vi "follow_angle.vi"() -> (3 "PID A":T2(graph)={"Setpoint"=-0.02930742489899981, "output"=0.018032836156553524, "dx/dt"=0.0})   [LabVIEW 2017]
uses:
  <vilib>/myRIO/Common/Instrument Driver Framework/myRIO v1.0/Encoder/typedefs/Encoder Signal Mode.ctl
  <vilib>/myRIO/Instrument Drivers/Onboard IO/Encoder/typedefs/Encoder Reference.ctl
  <vilib>/myRIO/Common/Instrument Driver Framework/Utilities/typedefs/myRIO Generic Hardware Reference.ctl
  <vilib>/myRIO/Common/Instrument Driver Framework/Utilities/typedefs/Hardware Version Enum.ctl
  <vilib>/myRIO/Common/Instrument Driver Framework/Utilities/typedefs/myRIO v1.0 Reference.ctl
  <vilib>/myRIO/Common/Instrument Driver Framework/Utilities/typedefs/Generic FPGA Reference.ctl
  <vilib>/myRIO/Common/Instrument Driver Framework/myRIO v1.0/Encoder/typedefs/Encoder Channels Enum.ctl
  <vilib>/myRIO/Common/Instrument Driver Framework/myRIO v1.0/Encoder/typedefs/Encoder Configuration v1.0.ctl
  <vilib>/userdefined/High Color/nirio_resource_hc.ctl
  <vilib>/myRIO/Common/Instrument Driver Framework/Utilities/vis/Is FPGA Ref Available.vi
  <vilib>/myRIO/Common/Instrument Driver Framework/myRIO v1.0/Encoder/vis/myRIO v1.1 Open Encoder.vi
  <vilib>/myRIO/Instrument Drivers/Onboard IO/Encoder/vis/Read.vi
  <vilib>/myRIO/Common/Instrument Driver Framework/Utilities/vis/Validate Channels.vi
  <vilib>/myRIO/Common/Instrument Driver Framework/myRIO v1.0/Encoder/vis/myRIO v1.0 Reserve Encoder.vi
  <vilib>/myRIO/Common/Instrument Driver Framework/myRIO v1.0/UART/vis/myRIO v1.0 Close UART.vi
  <vilib>/myRIO/Common/Instrument Driver Framework/myRIO v1.0/Encoder/vis/myRIO v1.0 Build MUX Configuration Encoder.vi
  <vilib>/myRIO/Common/Instrument Driver Framework/myRIO v1.0/Resource Manager/vis/myRIO v1.0 Reserve Channel List.vi
  <vilib>/myRIO/Common/Instrument Driver Framework/myRIO v1.0/Resource Manager/vis/myRIO v1.0 Create Configuration List.vi
  <vilib>/myRIO/Common/Instrument Driver Framework/myRIO v1.0/Resource Manager/vis/myRIO v1.0 Reserve Channel.vi
  <vilib>/myRIO/Common/Instrument Driver Framework/myRIO v1.0/Resource Manager/vis/myRIO v1.0 Unreserve Channel.vi
  <vilib>/myRIO/Common/Instrument Driver Framework/myRIO v1.0/Resource Manager/vis/myRIO v1.0 Build Mutex Name.vi
  <vilib>/Utility/VariantDataType/GetNumericInfo.vi
  <vilib>/Utility/error.llb/Error Cluster From Error Code.vi
  <vilib>/myRIO/Common/Instrument Driver Framework/myRIO v1.0/myRIO v1.1 Open.vi
  <vilib>/myRIO/Common/Instrument Driver Framework/Utilities/vis/IO Manager.vi
  <vilib>/myRIO/Common/Instrument Driver Framework/Utilities/vis/Configuration Manager.vi
  <vilib>/myRIO/Common/Instrument Driver Framework/myRIO v1.0/Resource Manager/vis/myRIO v1.0 Configure IO.vi
  <vilib>/myRIO/Common/Instrument Driver Framework/myRIO v1.0/myRIO v1.0 Close.vi
  <vilib>/myRIO/Common/Instrument Driver Framework/myRIO v1.0/Encoder/vis/myRIO v1.0 Configure Encoder.vi
  <vilib>/myRIO/Common/Instrument Driver Framework/myRIO v1.0/Encoder/vis/myRIO v1.0 Read Encoder.vi
  <vilib>/myRIO/Common/Instrument Driver Framework/Utilities/vis/FPGA Ref Manager.vi
  <vilib>/myRIO/Common/Instrument Driver Framework/myRIO v1.0/myRIO v1.0 Reset FPGA.vi
  <vilib>/myRIO/Common/Instrument Driver Framework/myRIO v1.0/IRQ/vis/myRIO v1.0 IRQ Info FGV.vi
  <vilib>/myRIO/Common/Instrument Driver Framework/myRIO v1.0/IRQ/vis/myRIO v1.0 Timer IRQ Info FGV.vi
  <vilib>/myRIO/Common/Instrument Driver Framework/myRIO v1.0/IRQ/vis/myRIO v1.0 ISR Agent.vi
  <vilib>/addons/control/pid/pid.llb/PID (DBL).vi
  <vilib>/myRIO/Express VI/Onboard IO/Encoder/Encoder Express VI.xnode
  <vilib>/myRIO/Instrument Drivers/Onboard IO/Encoder/vis/myRIO Encoder Open.xnode
  <vilib>/myRIO/Common/Instrument Driver Framework/myRIO v1.0/Encoder/typedefs/Encoder Count Direction Enum.ctl
  <vilib>/myRIO/Instrument Drivers/Utilities/Utilities.lvlib
  <vilib>/myRIO/Instrument Drivers/Onboard IO/Encoder/Encoder.lvlib
  <vilib>/addons/control/pid/NI_PID_pid.lvlib
panel:
  out "Angle":cluster{"Angle to Follow":dbl, dbl}(graph)={"Angle to Follow"=-9.27038626609442, -9.052560000004503}
  in  "Angle PIDS":T1={"proportional gain (Kc)"=0.05, "integral time (Ti, min)"=0.05, "derivative time (Td, min)"=0.0} {"derivative time (Td, min)" format="%.3f"; "integral time (Ti, min)" format="%.3f"; "proportional gain (Kc)" format="%.3f"}
  in  "Angle to Follow":dbl(slide)=-9.27038626609442 scale=-360.0..360.0
  in  "stop":bool
  in  "Speed":dbl(slide)=-0.015174506828527612 scale=-10.0..10.0
  out "OUTPUT B":dbl(slide) scale=-10.0..10.0
  out "OUTPUT A":dbl(slide) scale=-10.0..10.0
  out "PID B":T2(graph)={"Setpoint"=-0.0010415887580554149, "output"=-0.02086159598615355, "dx/dt"=0.0}
  out "Setpoint A":dbl(slide)=-0.02930742489899981 scale=-10.0..10.0
  out "Setpoint B":dbl(slide)=-0.0010415887580554149 scale=-10.0..10.0
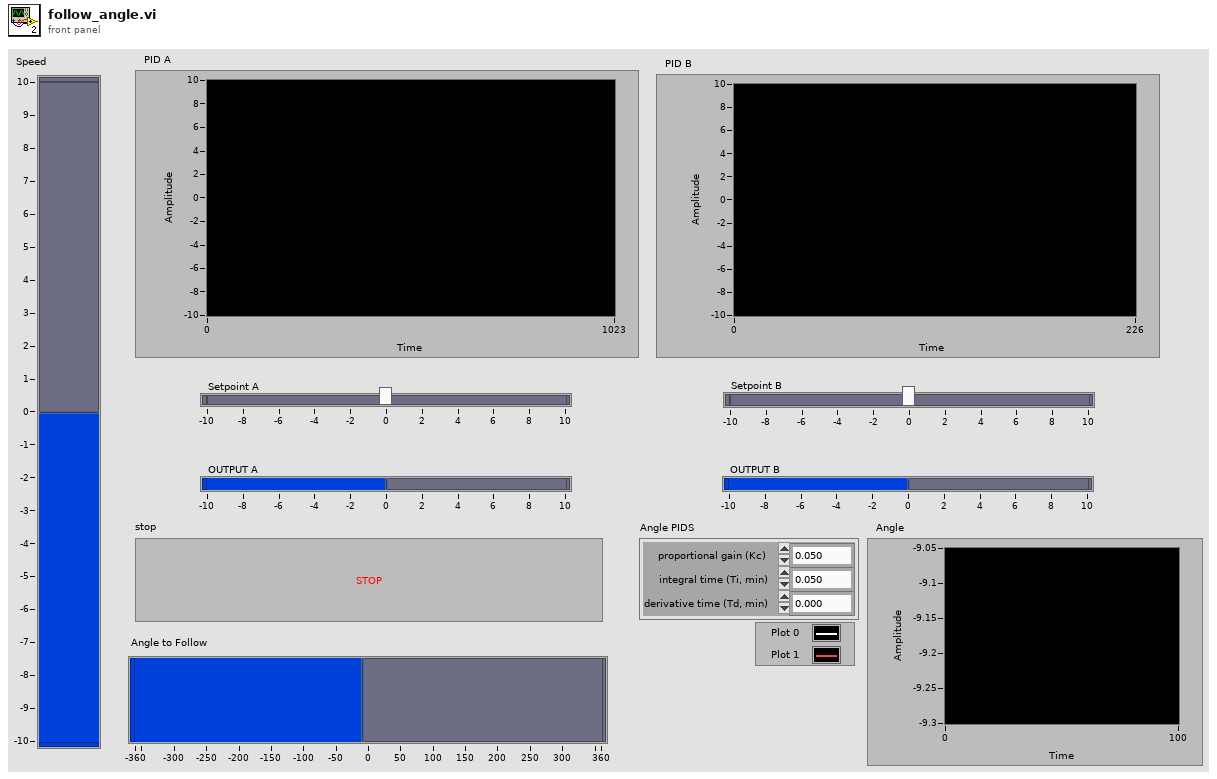
[diagram p1: front panel]
types:
  T1 = cluster{"proportional gain (Kc)":dbl, "integral time (Ti, min)":dbl, "derivative time (Td, min)":dbl}
  T2 = cluster{"Setpoint":dbl, "output":dbl, "dx/dt":dbl}
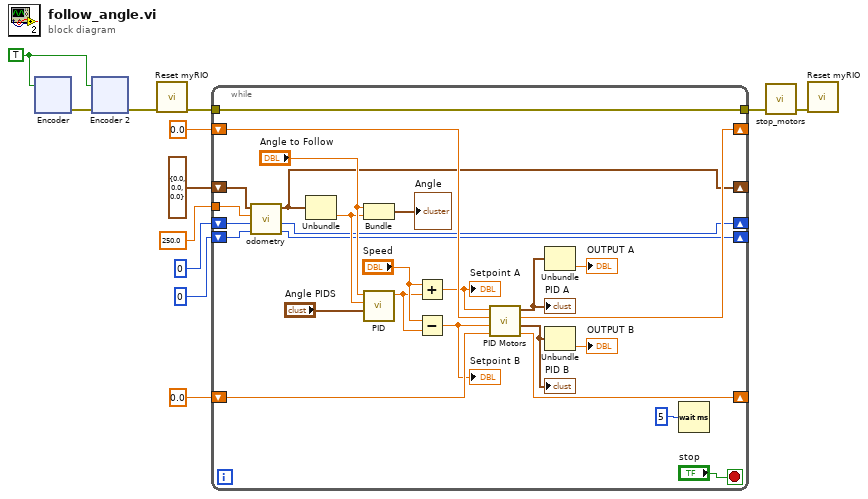
[diagram p0: block diagram]
diagram:
  w9 = TRUE
  n1 = xnode "Encoder"("Reset Counter"=w9) -> ("error out"=w10:errorcluster)  [unwired: 1 in, 3 out]
  n2 = xnode "Encoder 2"("error in (no error)"=w10, "Reset Counter"=w9) -> ("error out"=w11:errorcluster)  [unwired: 3 out]
  n3 = call <vilib>:"Reset myRIO.vi"("error in (no error)"=w11) -> ("error out"=w12:errorcluster)  [unwired: 10 in]
  n4 = while {
    tunnel: w12 -> [w33]
    shift-right: [w35] -> _
    shift-left: 0.0 ("output A") -> [w36]
    shift-right: [w38] -> _
    shift-left: 0.0 ("output B") -> [w37]
    tunnel: [w33] -> w5
    shift-right: [w19] -> _
    shift-left: 0 ("ENCA OUT") -> [w17]
    shift-right: [w18] -> _
    shift-left: 0 ("ENCB OUT") -> [w16]
    shift-right: [w15] -> _
    shift-left: cluster{dbl, dbl, dbl} {0.0, 0.0, 0.0} ("X, Y, BEARING") -> [w14]
    tunnel: 250.0 ("wheelbase") -> [w13]
    stop <- "stop" stop-if-true
    n5 = call "odometry.vi"("ENCB in"=w16, "ENCA in"=w17, "wheelbase"=w13, "Position"=w14) -> ("ENCB OUT"=w18:i32, "ENCA OUT"=w19:i32, "X, Y, BEARING"=w15:cluster{dbl, dbl, dbl})  [unwired: 4 in]
    n6 = Unbundle(w15) -> (w21:dbl)  [unwired: 2 out]
    n7 = Bundle("Angle to Follow"="Angle to Follow", w21) -> (→"Angle":cluster{"Angle to Follow":dbl, dbl})  [unwired: 1 in]
    n8 = call-poly <vilib>:"PID.vi"("PID gains"="Angle PIDS", "process variable"=w21, "setpoint"="Angle to Follow") -> ("output"=w27:dbl)  [unwired: 7 in, 1 out]
    n9 = Add(x="Speed", y=w27) -> (x+y=w23:dbl)
    "Setpoint A" <- w23
    n10 = Subtract(x="Speed", y=w27) -> (x-y=w24:dbl)
    "Setpoint B" <- w24
    n11 = call "PID Motors.vi"("input B"=w37, "Speed B"=w24, "input A"=w36, "Speed A"=w23) -> ("output B"=w38:dbl, "Speed B0"=w31:T2, "output A"=w35:dbl, "Speed A0"=w32:T2)
    "PID B" <- w31
    "PID A" <- w32
    n12 = Unbundle(w32) -> ("dx/dt"=→"OUTPUT A":dbl)  [unwired: 2 out]
    n13 = Unbundle(w31) -> ("dx/dt"=→"OUTPUT B":dbl)  [unwired: 2 out]
    n14 = Wait (ms)(milliseconds to wait=5 ("ENCB OUT")) -> ()  [unwired: 1 out]
  }
  n15 = call "stop_motors.vi"("error in (no error)"=w5) -> ("error out"=w6:errorcluster)  [unwired: 4 in]
  n16 = call <vilib>:"Reset myRIO.vi"("error in (no error)"=w6) -> ()  [unwired: 10 in, 1 out]
